vi "SRV_Parse Formula String.vi"(8 "error in (no error)":errorcluster, 11 "Formula":string="(1/(v+5))+20") -> (0 "error out":errorcluster, 2 "Parsed Formula":cluster{"Table":i32[][], "Y Values":dbl[]} {"Y Values" format="%.2f"})   [LabVIEW 2014]
doc: "Analyzes a string as a formula and produces two numeric arrays. These arrays can be used by the Eval Parsed Formula String VI.\n\nFormula must use \"v\" for the variable name (v is not case sensitive).\n\n\nAuthor: Mike Schultz (mschultz11711@gmail.com)"
uses:
  <vilib>/gmath/NI_Gmath.lvlib
panel:
  # "operator"
  # "register1"
  # "register2"
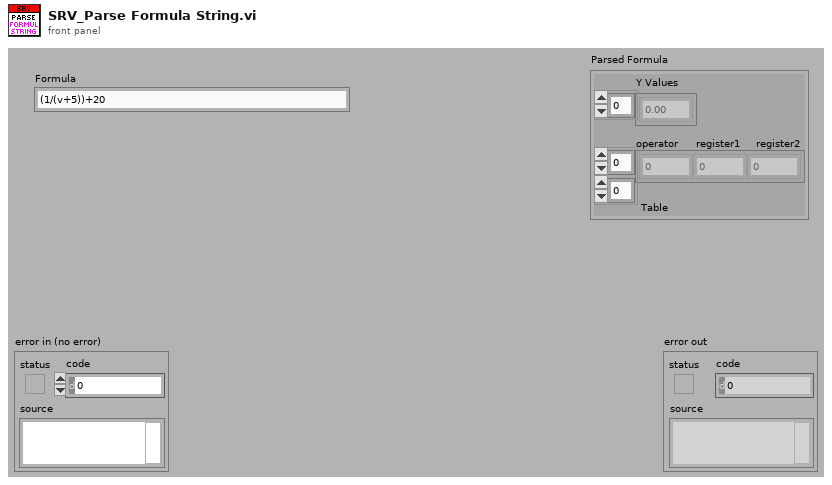
[diagram p1: front panel]
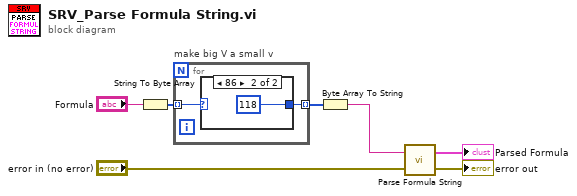
[diagram p0: block diagram]
diagram:
  n1 = String To Byte Array(string="Formula") -> (unsigned byte array=w6:u8[])
  n2 = for "make big V a small v" {
    tunnel: w6 -> [w9] mode=indexing
    tunnel: [w8] -> w3 mode=indexing
    n3 = case shown="86" w9 {
      selector: w9 -> [w10 _]
      tunnel: [w10 u8 118] -> w8
      frame Default {
      }
      frame 86 {
      }
    }
  }
  n4 = Byte Array To String(unsigned byte array=w3) -> (string=w1:string)
  n5 = call <vilib>:"Parse Formula String.vi"("error in (no error)"="error in (no error)", "formula"=w1) -> ("error out"=→"error out":errorcluster, "Parsed Formula"=→"Parsed Formula":cluster{"Table":i32[][], "Y Values":dbl[]})
